vi "Single_Read Index Set.vi"(9 "Default":sgl[](array[numeric]), 11 "Indices":i32[](array[numeric])) -> (1 "Values":sgl[](array[numeric]))   [LabVIEW 2016, in "CVT.lvlib" / "Current Value Table.lvlib"]
doc: "This VI reads a set of data as defined by the GetIndices function. This VI can provide an order of magnitude increase in performance over a normal index read for sufficiently large data sets."
uses:
  <vilib>/NI/Current Value Table/Current Value Table.lvlib
  <vilib>/NI/Current Value Table/Type Defs/Memory Commands.ctl
  <vilib>/NI/Current Value Table/DataTypes/Single_Memory Block.vi
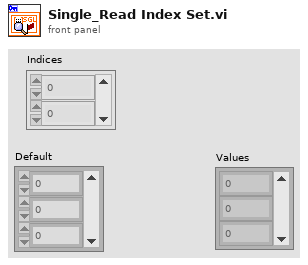
[diagram p1: front panel]
types:
  T1 = typedef "CVT.lvlib/Current Value Table.lvlib/Memory Commands.ctl" = enum16{"Init", "Add Data", "Read", "Read Group", "Read All", "Write", "Write Group", "Get Size"}
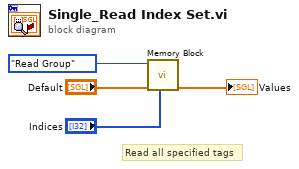
[diagram p0: block diagram]
diagram:
  # "Read all specified tags"
  n1 = call-poly <vilib>:"Memory Block.vi"("Group Indices"="Indices", "Data In"="Default", "Method"=Memory_Commands."Read Group") -> ("Group Data"=→"Values":sgl[])  [unwired: 6 in, 2 out]
